vi "Test Line Tracker Controller.vi"() -> ()   [LabVIEW 2026]
uses:
  Line Tracker/Line Tracker/Tracking Values.ctl
  <vilib>/ActorFramework/Message Enqueuer/Message Enqueuer.lvclass/Message Enqueuer.ctl
  <vilib>/ActorFramework/Message Enqueuer/Enqueue.vi
  Line Tracker/Line Tracker/Line Tracker.lvclass
  usr/local/natinst/LabVIEW-2026-64/vi.lib/ActorFramework/Actor/Actor.lvclass
  <vilib>/ActorFramework/Stop Msg/Stop Msg.lvclass
  usr/local/natinst/LabVIEW-2026-64/vi.lib/ActorFramework/Message/Message.lvclass
  <vilib>/ActorFramework/Message Priority Queue/Priority Enqueue.vi
  <vilib>/ActorFramework/Actor/Actor.lvclass
  CTI-Grove/Examples/Sourcecode/cti-drivers-lv-visa-simple/Examples/Driver/CTIPicoVISA.lvlib
panel:
  out "Tracking Values":T1
  out "error out":errorcluster
  in  "stop":bool
  in  "VISA resource name":refnum<visa-resource-name>
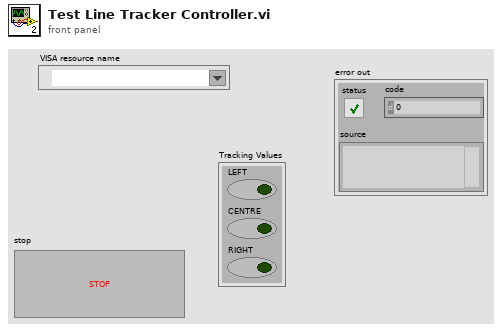
[diagram p1: front panel]
types:
  T1 = typedef "Tracking Values.ctl" = cluster{"LEFT":bool, "CENTRE":bool, "RIGHT":bool}
  T2 = typedef "User Events.ctl" = cluster{"Tracking Values":refnum<user-event>, "Stop":refnum<user-event>}
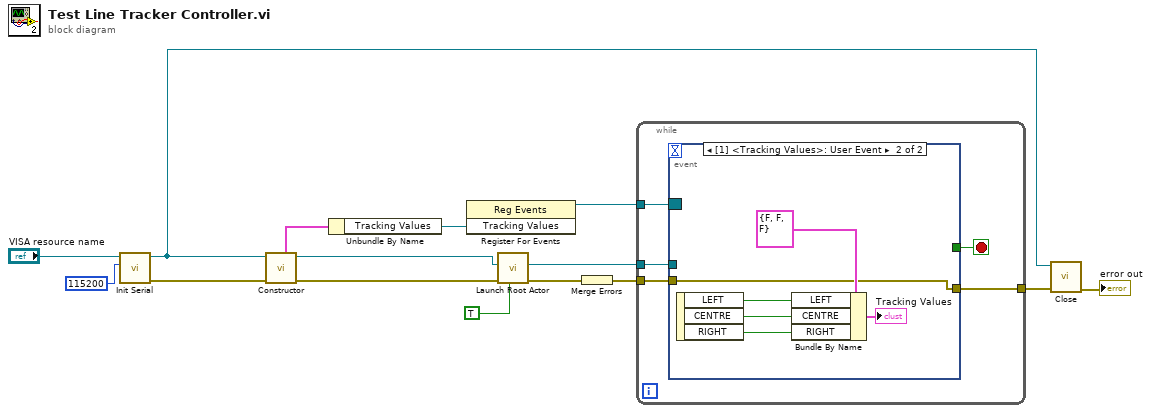
[diagram p0: block diagram]
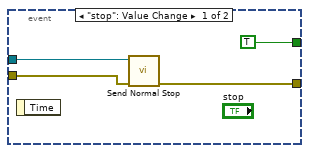
[diagram p2: hidden frame]
diagram:
  n1 = call "Init Serial.vi"("Baud (115200)"=u32 115200, "VISA resource name in"="VISA resource name") -> ("error out"=w12:errorcluster, "VISA resource name Out"=w7:refnum<visa-resource-name>)  [unwired: 7 in, 1 out]
  n2 = call "Constructor.vi"("error in (no error)"=w12, "VISA resource name"=w7) -> ("error out"=w5:errorcluster, "Line Tracker out"=w6:refnum<class "Line Tracker.lvclass">, "User Events"=w3:T2)  [unwired: 7 in]
  n3 = Unbundle By Name(w3) -> ("Tracking Values"=w1:refnum<user-event>)
  n4 = register-events(w1) -> (reference out=w2:refnum<event-registration>)  [unwired: 2 in, 1 out]
  n5 = call <vilib>:"Launch Root Actor.vi"("Open Actor Core front panel? (F)"=TRUE, "error in (no error)"=w5, "Actor"=w6) -> ("error out"=w11:errorcluster, "Actor's Enqueuer"=w15:refnum<class "Message Enqueuer.lvclass">)  [unwired: 7 in]
  n6 = Merge Errors(w11) -> (w10:errorcluster)
  n7 = while {
    tunnel: w15 -> [w20]
    tunnel: [w18] -> w9
    tunnel: w10 -> [w17]
    tunnel: w2 -> [w16]
    stop <- w19 stop-if-true
    n8 = event shown="[1] <Tracking Values>: User Event" {
      selector: w16 -> [_ _]
      dyn-events: _ -> [_ _]
      timeout: _ -> [_ _]
      tunnel: w20 -> [w24 _]
      tunnel: [w23 w25] -> w18
      tunnel: [TRUE _] -> w19
      tunnel: w17 -> [w21 w25]
      event "stop": Value Change {
        n9 = event-data() -> ()  [unwired: 1 in, 1 out]
        n10 = call <vilib>:"Send Normal Stop.vi"("error in (no error)"=w21, "Message Enqueuer"=w24) -> ("error out"=w23:errorcluster)  [unwired: 9 in]
      }
      event User Event {
        n11 = event-data() -> ("LEFT"=w29:bool, "CENTRE"=w27:bool, "RIGHT"=w28:bool)  [unwired: 1 in]
        n12 = Bundle By Name(cluster=T1 {"LEFT"=FALSE, "CENTRE"=FALSE, "RIGHT"=FALSE} ("Cluster"), "LEFT"=w29, "CENTRE"=w27, "RIGHT"=w28) -> (→"Tracking Values":T1)
      }
    }
  }
  n13 = call "Close.vi"("error in (no error)"=w9, "VISA resource name in"=w7) -> ("error out"=→"error out":errorcluster)  [unwired: 9 in]
